vi "Read Single Meas.vi"(8 "error in (no error)":errorcluster, 11 "Agilent 34401A in":refnum<class "Agilent 34401A.lvclass">) -> (0 "error out":errorcluster, 2 "Value":dbl, 3 "Agilent 34401A out":refnum<class "Agilent 34401A.lvclass">)   [LabVIEW 2021, in "DMM.lvlib" / "Agilent 34401A.lvclass"]
uses:
  Agilent 34401A.lvclass
  Agilent 34401A.lvclass/Agilent 34401A.ctl
  <instrlib>/Agilent 34401/Public/Data/Read (Single Point).vi
  <instrlib>/Agilent 34401/Agilent 34401.lvlib
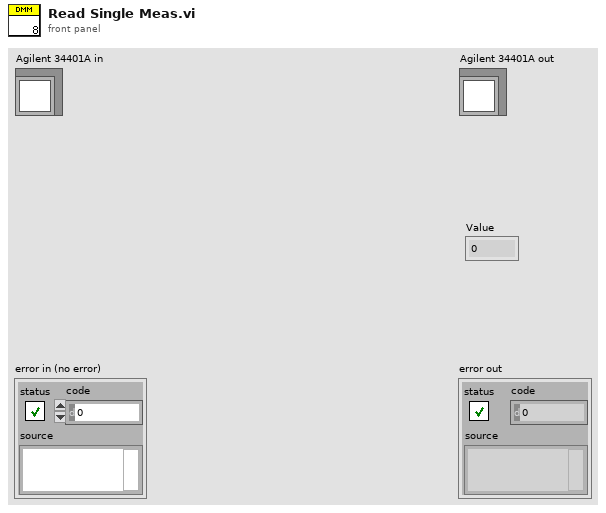
[diagram p1: front panel]
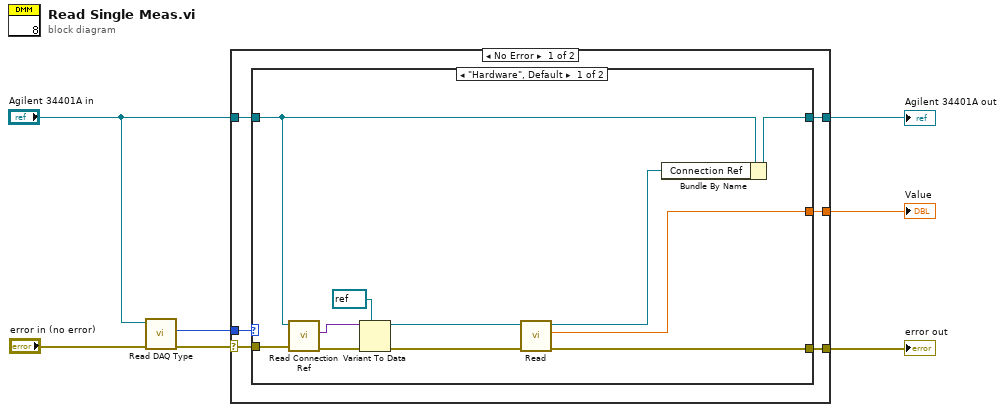
[diagram p0: block diagram]
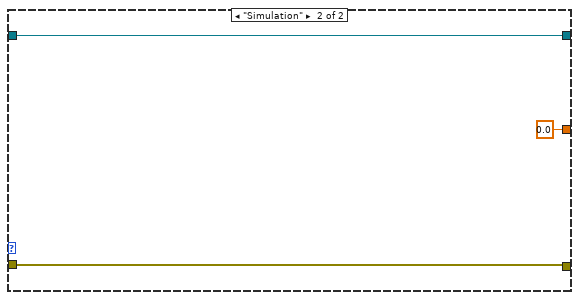
[diagram p2: hidden frame]
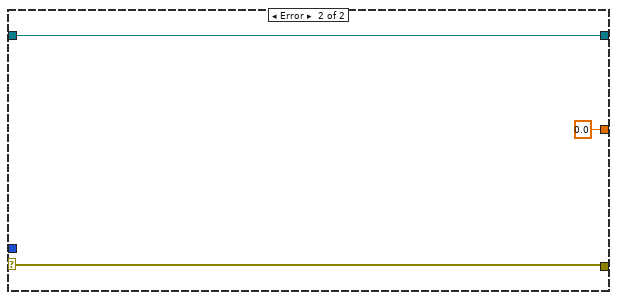
[diagram p3: hidden frame]
diagram:
  n1 = call-dynamic "Read DAQ Type.vi"("error in (no error)"="error in (no error)", "Agilent 34401A in"="Agilent 34401A in") -> ("error out"=w6:errorcluster, "DAQ Type"=w5:enum16{"Hardware", "Simulation"})  [unwired: 7 in, 1 out]
  n2 = case shown="No Error" w6 {
    selector: w6 -> [w11 w28]
    tunnel: w5 -> [w13 _]
    tunnel: "Agilent 34401A in" -> [w12 w30]
    tunnel: [w10 w30] -> w3
    tunnel: [w9 w28] -> w2
    tunnel: [w8 0.0 ("Measurement")] -> w1
    frame No Error {
      n3 = case shown="\"Hardware\", Default" w13 {
        tunnel: w12 -> [w18 w27]
        tunnel: w11 -> [w24 w26]
        tunnel: [w16 w27] -> w10
        tunnel: [w17 w26] -> w9
        tunnel: [w14 0.0 ("Measurement")] -> w8
        frame "Hardware", Default {
          n4 = call-dynamic "Read Connection Ref.vi"("error in (no error)"=w24, "Agilent 34401A in"=w18) -> ("error out"=w23:errorcluster, "Connection Ref"=w22:variant)  [unwired: 7 in, 1 out]
          n5 = Variant To Data(error in=w23, type=refnum<visa-resource-name> refnum ("VISA resource name"), Variant=w22) -> (data=w20:refnum<visa-resource-name>, error out=w19:errorcluster)
          n6 = call-poly <instrlib>:"Read.vi"("error in (no error)"=w19, "VISA resource name"=w20) -> ("error out"=w17:errorcluster, "Measurement"=w14:dbl, "VISA resource name out"=w15:refnum<visa-resource-name>)  [unwired: 7 in]
          n7 = Bundle By Name(cluster=w18, "Connection Ref"=w15) -> (w16:refnum<class "Agilent 34401A.lvclass">)
        }
        frame "Simulation" {
        }
      }
    }
    frame Error {
    }
  }
  "error out" <- w2
  "Agilent 34401A out" <- w3
  "Value" <- w1
